vi "GetOwningPane__LCR.vi"(8 "error in (no error)":errorcluster, 11 "Control Reference":refnum<vi> caption="Control") -> (0 "error out":errorcluster, 2 "Owning Pane":refnum<vi>)   [LabVIEW 2011, in "BooleanXControl__LCR.xctl"]
doc: "VI to get the owing Pane of a given control"
uses:
  BooleanXControl__LCR.xctl
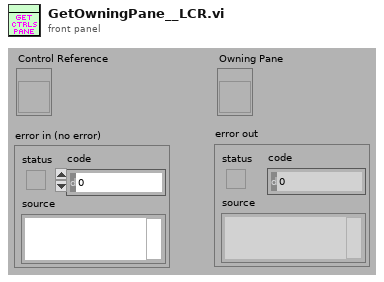
[diagram p1: front panel]
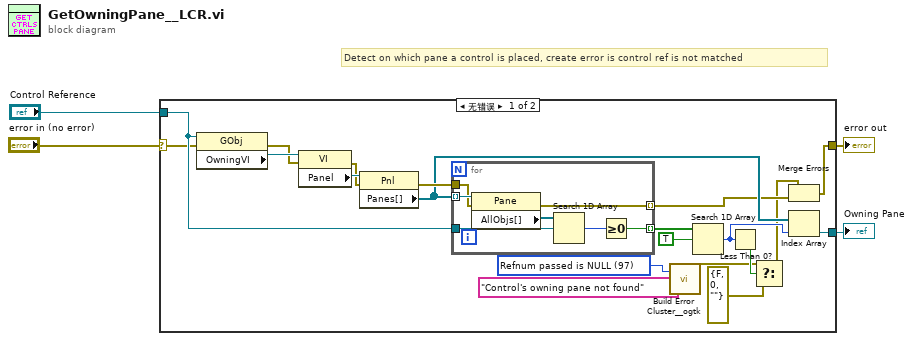
[diagram p0: block diagram]
diagram:
  # "Detect on which pane a control is placed, create error is control ref is not matched"
  n1 = case shown="无错误" "error in (no error)" {
    selector: "error in (no error)" -> [w14 w32]
    tunnel: [w16 _] -> w4
    tunnel: "Control Reference" -> [w15 _]
    tunnel: [w13 w32] -> w1
    frame No Error {
      w11 = 97 items=["No error", "Argument error", "Memory is full", "Out of zone", "End of file", "File already open", "Generic file I/O error", "File not found", "File permission error", "Disk is full", "Duplicate path", "Too many files open", "System feature not enabled", "Resource file not found", "Cannot add resource", "Resource not found", "Image not found", "Image memory error", "Pen does not exist", "Config type invalid", "Config token not found", "Config parse error", "Config memory error", "Bad external code format", "Bad external code offset", "External code not present", "Null window", "Destroy window error", "Null menu", "Print aborted", "Bad print record", "Print driver error", "Windows error during printing", "Memory error during printing", "Print dialog error", "Generic print error", "Invalid device refnum", "Device not found", "Device parameter error", "Device unit error", "Cannot open device", "Device call aborted", "Generic error", "Cancelled by user", "Object ID too low", "Object ID too high", "Object not in heap", "Unknown heap", "Unknown object (invalid DefProc)", "Unknown object (DefProc not in table)", "Message out of range", "Invalid (null) method", "Unknown message", "Manager call not supported", "Bad address", "Network operation in progress", "Network operation timed out", "Connection is busy", "Network attribute not supported", "Network error", "Address in use", "System out of memory", "Connection aborted", "Connection refused", "Not connected", "Already connected", "Connection closed", "Initialization error (interapplication manager)", "Bad occurrence", "Wait on unbound occurrence handler", "Occurrence queue overflow", "Datalog type conflict", "Unused", "Unrecognized type (interapplication manager)", "Memory corrupt", "Failed to make temporary DLL", "Old CIN version", "Drag socket not found", "Failed to load drop-object", "Failed to register OLE object", "Failed to release OLE object", "Format specifier type mismatch", "Unknown format specifier", "Too few format specifiers", "Too many format specifiers", "Scan failed", "Newer CIN version", "Error converting to variant", "Runtime menu error", "Password tampered", "Variant attribute not found", "Incompatible variant data type", "Event data is not available", "Event Store is not present", "Occurrence is not found", "Event Queue is not created", "Event info is not available", "Refnum passed is NULL", "Error retrieving Class GUID", "Error retrieving CoClass GUID", "Error retrieving TypeLib GUID.", "Bad built application magic bytes.", "Specific driver is different from the specific driver associated with the Logical Name.", "There is no session opened to the class driver.", "Max Error", "MAX - Error with config objects", "MAX - Error loading configuration", "MAX - Group not supported"]
      n2 = property class="GObj"(reference=w15, error in=w14) -> (error out=w22:errorcluster, "OwningVI"=w24:refnum<vi>)  [unwired: 1 out]
      n3 = property class="VI"(reference=w24, error in=w22) -> (error out=w21:errorcluster, "Panel"=w23:refnum<vi>)  [unwired: 1 out]
      n4 = property class="Pnl"(reference=w23, error in=w21) -> (error out=w20:errorcluster, "Panes[]"=w17:refnum<vi>[])  [unwired: 1 out]
      n5 = for {
        tunnel: w17 -> [w31] mode=indexing
        tunnel: w20 -> [w30]
        tunnel: w15 -> [w28]
        tunnel: [w26] -> w19 mode=indexing
        tunnel: [w25] -> w12 mode=indexing
        n6 = property class="Pane"(reference=w31, error in=w30) -> (error out=w25:errorcluster, "AllObjs[]"=w29:refnum<vi>[])  [unwired: 1 out]
        n7 = Search 1D Array(1D array=w29, element=w28) -> (index of element=w27:i32)  [unwired: 1 in]
        n8 = Greater Or Equal To 0?(x=w27) -> (x >= 0?=w26:bool)
      }
      n9 = call <userlib>:"Build Error Cluster__ogtk.vi"("String to Prepend to source (\"\")"="Control's owning pane not found" ("String to Prepend to source (\"\")"), "code"=w11) -> ("error out"=w7:errorcluster)
      n10 = Search 1D Array(1D array=w19, element=TRUE) -> (index of element=w9:i32)  [unwired: 1 in]
      n11 = Less Than 0?(x=w9) -> (x < 0?=w8:bool)
      n12 = Select(t=w7, s=w8, f=errorcluster {"status"=FALSE, "code"=0, "source"=""}) -> (s? t:f=w5:errorcluster)
      n13 = Merge Errors(w5, w12) -> (w13:errorcluster)
      n14 = Index Array(array=w17, index=w9) -> (element=w16:refnum<vi>)
    }
    frame Error {
    }
  }
  "Owning Pane" <- w4
  "error out" <- w1
